vi "Init - Add NTeeth and FullCustom.vi"(8 "error in (no error)":errorcluster, 9 "FullyCustom Components":T3[](array[typedef]), 10 "NTeeth Components":T2[](array[typedef]), 11 "Crank Cams Page in":T1 format="%.0x") -> (0 "error out":errorcluster, 3 "Crank Cams Page out":T1 format="%.0x")   [LabVIEW 2011, in "Engine Sim System Explorer.lvlib"]
uses:
  Engine Sim System Explorer.lvlib
  TypeDefs/FullyCustomComp.ctl
  Shared/FullyCustomCommMode.ctl
  TypeDefs/FullyCustomProfilesComp.ctl
  TypeDefs/NTeethComp.ctl
  <vilib>/NI Veristand/Custom Device API/Custom Device Item Ref.ctl
  <vilib>/NI Veristand/Custom Device API/Custom Device Channel.ctl
  <vilib>/NI Veristand/Custom Device API/Custom Device Channel Type.ctl
  Shared/Engine Simulation Global.vi
  <vilib>/NI Veristand/Custom Device API/Custom Device API.lvlib
  Engine Simulation Shared.lvlib
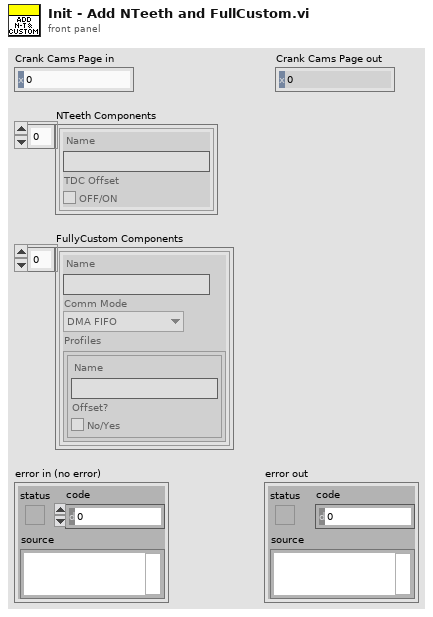
[diagram p1: front panel]
types:
  T1 = typedef "Custom Device API.lvlib/Custom Device Item Ref.ctl" = u64
  T2 = typedef "Engine Sim System Explorer.lvlib/NTeethComp.ctl" = cluster{"Name":string, "TDC Offset":bool}
  T3 = typedef "Engine Sim System Explorer.lvlib/FullyCustomComp.ctl" = cluster{"Name":string, "Comm Mode":T4, "Profiles":T5[]}
  T4 = typedef "Engine Simulation Shared.lvlib/FullyCustomCommMode.ctl" = enum16{"DMA FIFO", "FP Data Transfer"}
  T5 = typedef "Engine Sim System Explorer.lvlib/FullyCustomProfilesComp.ctl" = cluster{"Name":string, "Offset?":bool}
  T6 = typedef "Custom Device API.lvlib/Custom Device Channel.ctl" = cluster{"Type":T7, "Units":string, "Default Value":dbl, "Faultable":bool, "Scalable":bool}
  T7 = typedef "Custom Device API.lvlib/Custom Device Channel Type.ctl" = enum16{"Input", "Output"}
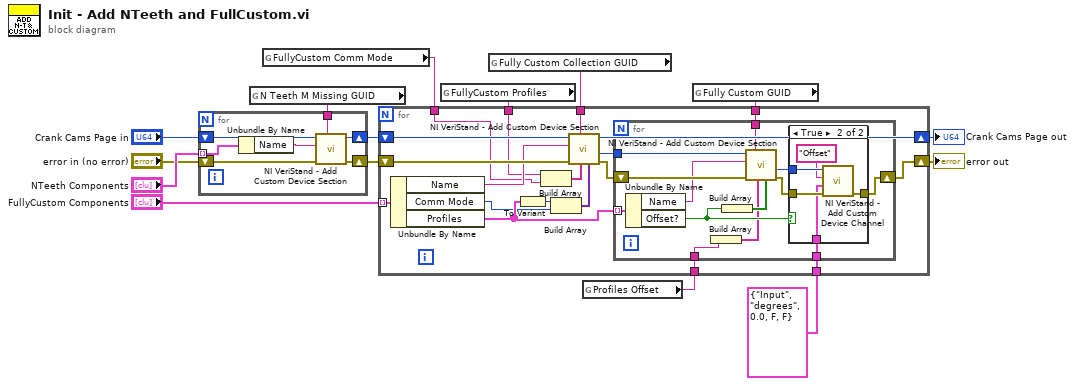
[diagram p0: block diagram]
diagram:
  n1 = global read "Engine Simulation Global.vi" "N Teeth M Missing GUID"() -> (w5:string)
  n2 = for {
    tunnel: "NTeeth Components" -> [w22] mode=indexing
    shift-right: [w21] -> w9
    shift-left: "error in (no error)" -> [w20]
    tunnel: w5 -> [w19]
    shift-right: [w16] -> w8
    shift-left: "Crank Cams Page in" -> [w18]
    n3 = Unbundle By Name(w22) -> ("Name"=w17:string)
    n4 = call <vilib>:"NI VeriStand - Add Custom Device Section.vi"("GUID (Default Section)"=w19, "error in (no error)"=w20, "Section Name"=w17, "Parent Ref in"=w18) -> ("error out"=w21:errorcluster, "Parent Ref out"=w16:T1)  [unwired: 4 in, 2 out]
  }
  n5 = global read "Engine Simulation Global.vi" "FullyCustom Comm Mode"() -> (w15:string)
  n6 = global read "Engine Simulation Global.vi" "FullyCustom Profiles"() -> (w13:string)
  n7 = global read "Engine Simulation Global.vi" "Fully Custom Collection GUID"() -> (w7:string)
  n8 = global read "Engine Simulation Global.vi" "Profiles Offset"() -> (w12:string)
  n9 = global read "Engine Simulation Global.vi" "Fully Custom GUID"() -> (w6:string)
  n10 = for {
    shift-right: [w41] -> w10
    shift-left: w9 -> [w40]
    tunnel: w7 -> [w38]
    tunnel: w6 -> [w37]
    tunnel: w12 -> [w36]
    tunnel: T6 {"Type"=enum."Input", "Units"="degrees", "Default Value"=0.0, "Faultable"=FALSE, "Scalable"=FALSE} ("Channel") -> [w35]
    shift-right: [w28] -> w1
    shift-left: w8 -> [w39]
    tunnel: "FullyCustom Components" -> [w27] mode=indexing
    tunnel: w13 -> [w26]
    tunnel: w15 -> [w24]
    n11 = Unbundle By Name(w27) -> ("Name"=w34:string, "Comm Mode"=w23:T4, "Profiles"=w25:T5[])
    n12 = To Variant(anything=w25) -> (Variant=w32:variant)
    n13 = Build Array(w26, w24) -> (w31:string[])
    n14 = Build Array(w32, w23) -> (w33:variant[])
    n15 = call <vilib>:"NI VeriStand - Add Custom Device Section.vi"("Property Values"=w33, "Property names"=w31, "GUID (Default Section)"=w38, "error in (no error)"=w40, "Section Name"=w34, "Parent Ref in"=w39) -> ("error out"=w29:errorcluster, "Section Ptr"=w30:T1, "Parent Ref out"=w28:T1)  [unwired: 2 in, 1 out]
    n16 = for {
      tunnel: w30 -> [w54]
      tunnel: w25 -> [w52] mode=indexing
      tunnel: w37 -> [w50]
      shift-right: [w45] -> w41
      shift-left: w29 -> [w53]
      tunnel: w36 -> [w43]
      tunnel: w35 -> [w44]
      n17 = Unbundle By Name(w52) -> ("Name"=w51:string, "Offset?"=w47:bool)
      n18 = Build Array(w43) -> (w42:string[])
      n19 = Build Array(w47) -> (w46:bool[])
      n20 = call <vilib>:"NI VeriStand - Add Custom Device Section.vi"("Property Values"=w46, "Property names"=w42, "GUID (Default Section)"=w50, "error in (no error)"=w53, "Section Name"=w51, "Parent Ref in"=w54) -> ("error out"=w48:errorcluster, "Section Ptr"=w49:T1)  [unwired: 2 in, 2 out]
      n21 = case shown="True" w47 {
        tunnel: w49 -> [_ w60]
        tunnel: w48 -> [w55 w59]
        tunnel: [w55 w58] -> w45
        tunnel: w44 -> [_ w57]
        frame False {
        }
        frame True {
          n22 = call <vilib>:"NI VeriStand - Add Custom Device Channel.vi"("error in (no error)"=w59, "Channel"=w57, "Channel Name"="Offset" ("String"), "Parent Ref in"=w60) -> ("error out"=w58:errorcluster)  [unwired: 4 in, 3 out]
        }
      }
    }
  }
  "error out" <- w10
  "Crank Cams Page out" <- w1
